vi "启动整机测试 (子VI).vi"   [LabVIEW 2016]
uses:
  PLC/PLC.lvlib
types:
  T1 = enum32{"Bad", "Idle", "Run top level", "Running"}
  T2 = cluster{"氨氮":bool, "总磷":bool, "总氮":bool, "多参数":bool, "CODMn":bool, "CODcr":bool, "超标留样":bool}
  T3 = cluster{"测试模式":enum16{"正常测试", "集成干预"}, "参数启用":cluster{"氨氮":bool, "总磷":bool, "总氮":bool, "多参数":bool, "CODMn":bool, "CODcr":bool, "超标留样":bool}}
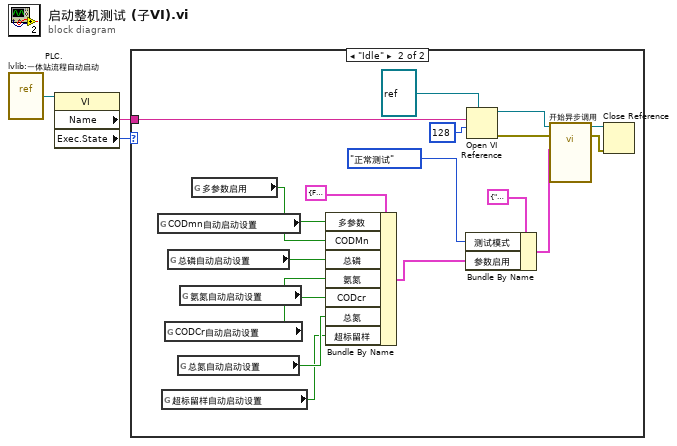
[diagram p0: block diagram]
diagram:
  n1 = vi-ref "PLC.lvlib:一体站流程自动启动.vi"() -> (w2:refnum<vi>)
  n2 = property class="VI"(reference=w2) -> ("Name"=w3:string, "Exec.State"=w1:T1)  [unwired: 1 in, 2 out]
  n3 = case shown="\"Idle\"" w1 {
    tunnel: w3 -> [_ w16]
    frame "Bad", Default {
    }
    frame "Idle" {
      n4 = global read "系统设置全局变量.vi" "CODmn自动启动设置"() -> (w14:bool)
      n5 = global read "系统设置全局变量.vi" "超标留样自动启动设置"() -> (w5:bool)
      n6 = global read "系统设置全局变量.vi" "CODCr自动启动设置"() -> (w11:bool)
      n7 = global read "系统设置全局变量.vi" "总磷自动启动设置"() -> (w13:bool)
      n8 = global read "系统设置全局变量.vi" "总氮自动启动设置"() -> (w10:bool)
      n9 = global read "系统设置全局变量.vi" "氨氮自动启动设置"() -> (w12:bool)
      n10 = global read "系统设置全局变量.vi" "多参数启用"() -> (w15:bool)
      n11 = Bundle By Name(cluster=T2 {"氨氮"=FALSE, "总磷"=FALSE, "总氮"=FALSE, "多参数"=FALSE, "CODMn"=FALSE, "CODcr"=FALSE, "超标留样"=FALSE} ("参数启用"), "多参数"=w15, "CODMn"=w14, "总磷"=w13, "氨氮"=w12, "CODcr"=w11, "总氮"=w10, "超标留样"=w5) -> (w4:T2)
      n12 = Bundle By Name(cluster=T3 {"测试模式"=enum."正常测试", "参数启用"={"氨氮"=FALSE, "总磷"=FALSE, "总氮"=FALSE, "多参数"=FALSE, "CODMn"=FALSE, "CODcr"=FALSE, "超标留样"=FALSE}} ("参数"), "测试模式"=enum16{"正常测试", "集成干预"}."正常测试", "参数启用"=w4) -> (w8:T3)
      n13 = Open VI Reference(type specifier VI Refnum (for type only)=refnum<vi> refnum, vi path=w16, options=128 ("选项")) -> (vi reference=w18:refnum<vi>, error out=w21:errorcluster)  [unwired: 3 in]
      n14 = call-by-ref "开始异步调用"(reference=w18, error in=w21, "参数"=w8) -> (reference out=w20:refnum<vi>, error out=w22:errorcluster)  [unwired: 11 in]
      n15 = Close Reference(reference=w20, error in (no error)=w22) -> ()  [unwired: 1 out]
    }
  }
